vi "Vision Processing.vi"(4 "error in (no error)":errorcluster, 7 "Image Size":T1=enum."320x240") -> ()   [LabVIEW 2017]
doc: "This VI runs in parallel to other tasks. It gets images from the camera, processes them for color or shape and use that information to affect robot behavior."
uses:
  <vilib>/Rock Robotics/WPI/Camera/WPI_CameraImageSize.ctl
  <vilib>/Rock Robotics/WPI/Camera/WPI_CameraWhite Balance Values.ctl
  <vilib>/Rock Robotics/WPI/Camera/WPI_CameraExposure Values.ctl
  <vilib>/Rock Robotics/WPI/Camera/WPI_CameraFrameRate.ctl
  Robot Global Data.vi
  <vilib>/vision/NI_Vision_Development_Module.lvlib
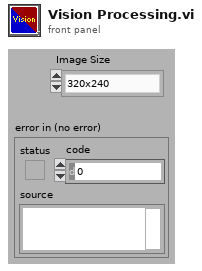
[diagram p1: front panel]
types:
  T1 = typedef "WPI_CameraImageSize.ctl" = enum16{"640x480", "320x240", "160x120", "Custom"}
  T2 = typedef "WPI_CameraFrameRate.ctl" = u32
  T3 = typedef "WPI_CameraExposure Values.ctl" = enum16{"Auto", "Flicker-free 50 Hz", "Flicker-free 60 Hz", "Hold current", "Custom"}
  T4 = typedef "WPI_CameraWhite Balance Values.ctl" = enum16{"Auto", "Fixed indoor", "Fixed outdoor 1", "Fixed outdoor 2", "Fixed fluorescent 1", "Fixed fluorescent 2", "Hold current", "Custom"}
  T5 = typedef "Image Type" = u32
  T6 = typedef "WPI_CameraDevRef.ctl" = cluster{"Camera Address":string, "CameraStatus":errorcluster}
  T7 = typedef "IMAQ Image.ctl" = refnum<image>
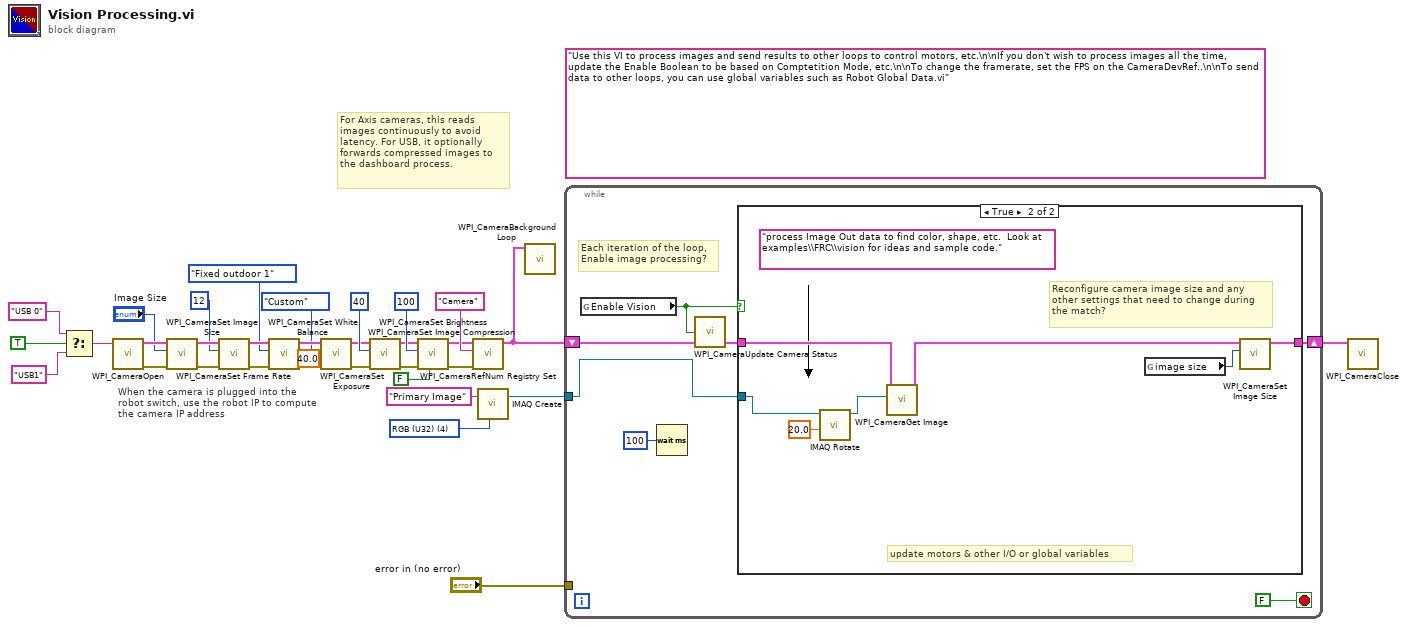
[diagram p0: block diagram]
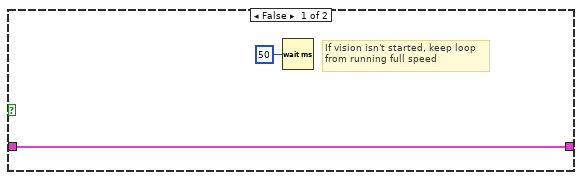
[diagram p2: hidden frame]
diagram:
  (unwired) "Use this VI to process images and send results to other loops to control motors, etc.\n\nIf you don't wish to process images all the time, update the Enable Boolean to be based on Comptetition Mode, etc.\n\nTo change the framerate, set the FPS on the CameraDevRef..\n\nTo send data to other loops, you can use global variables such as Robot Global Data.vi"
  w33 = T5 4 items=["Grayscale (U8)", "Grayscale (I16)", "Grayscale (SGL)", "Complex (CSG)", "RGB (U32)", "HSL (U32)", "RGB (U64)"] ("Image Type")
  # "When the camera is plugged into the\nrobot switch, use the robot IP to compute\nthe camera IP address"
  # "For Axis cameras, this reads\nimages continuously to avoid\nlatency. For USB, it optionally\nforwards compressed images to\nthe dashboard process."
  n1 = Select(t="USB 0" ("format string"), s=TRUE ("dot notation? (F)"), f="USB1" ("format string")) -> (s? t:f=w4:string)
  n2 = call <vilib>:"WPI_CameraOpen.vi"("Camera Address"=w4) -> ("error out"=w21:errorcluster, "CameraDevRef"=w22:T6)  [unwired: 1 in, 8 out]
  n3 = call <vilib>:"WPI_CameraSet Image Size.vi"("error in (no error)"=w21, "Image Size"="Image Size", "CameraDevRef"=w22) -> ("error out"=w20:errorcluster, "CameraDevRef Out"=w23:T6)  [unwired: 1 in, 6 out]
  n4 = call <vilib>:"WPI_CameraSet Frame Rate.vi"("error in (no error)"=w20, "Frame Rate (fps)"=T2 12, "CameraDevRef"=w23) -> ("error out"=w19:errorcluster, "CameraDevRef Out"=w25:T6)  [unwired: 7 out]
  n5 = call <vilib>:"WPI_CameraSet White Balance.vi"("error in (no error)"=w19, "White Balance"=WPI_CameraWhite_Balance_Values."Fixed outdoor 1", "CameraDevRef"=w25) -> ("error out"=w18:errorcluster, "CameraDevRef Out"=w24:T6)  [unwired: 1 in, 6 out]
  n6 = call <vilib>:"WPI_CameraSet Exposure.vi"("error in (no error)"=w18, "Exposure (%)"=40.0, "Exposure"=WPI_CameraExposure_Values."Custom", "CameraDevRef"=w24) -> ("error out"=w17:errorcluster, "CameraDevRef Out"=w27:T6)  [unwired: 6 out]
  n7 = call <vilib>:"WPI_CameraSet Image Compression.vi"("error in (no error)"=w17, "Compression"=40, "CameraDevRef"=w27) -> ("error out"=w16:errorcluster, "CameraDevRef Out"=w26:T6)  [unwired: 7 out]
  n8 = call <vilib>:"WPI_CameraSet Brightness.vi"("Force"=FALSE, "error in (no error)"=w16, "Brightness"=100, "CameraDevRef"=w26) -> ("error out"=w14:errorcluster, "CameraDevRef Out"=w15:T6)  [unwired: 6 out]
  n9 = call <vilib>:"WPI_CameraRefNum Registry Set.vi"("error in (no error)"=w14, "refnum name"="Camera", "CameraDevRef"=w15) -> ("CameraDevRef"=w10:T6)  [unwired: 1 in, 7 out]
  n10 = call "IMAQ Create"("Image Name"="Primary Image", "Image Type"=w33) -> ("New Image"=w31:T7)  [unwired: 2 in, 2 out]
  n11 = call <vilib>:"WPI_CameraBackground Loop.vi"("CameraDevRef"=w10) -> ()  [unwired: 11 in]
  n12 = while {
    shift-right: [w39] -> w8
    shift-left: w10 -> [w38]
    tunnel: w31 -> [w35]
    tunnel: "error in (no error)" -> [_]
    stop <- FALSE stop-if-true
    # "Each iteration of the loop,\nEnable image processing?"
    n13 = global read "Robot Global Data.vi" "Enable Vision"() -> (w36:bool)
    n14 = Wait (ms)(milliseconds to wait=u32 100) -> ()  [unwired: 1 out]
    n15 = call <vilib>:"WPI_CameraUpdate Camera Status.vi"("CameraDevRef In"=w38, "Enable Vision"=w36) -> ("CameraDevRef Out"=w37:T6)  [unwired: 3 in]
    n16 = case shown="True" w36 {
      tunnel: w35 -> [_ w45]
      tunnel: [w42 w49] -> w39
      tunnel: w37 -> [w42 w47]
      frame False {
        # "If vision isn't started, keep loop\nfrom running full speed"
        n17 = Wait (ms)(milliseconds to wait=u32 50) -> ()  [unwired: 1 out]
      }
      frame True {
        (unwired) "process Image Out data to find color, shape, etc.  Look at examples\\FRC\\vision for ideas and sample code."
        # "update motors & other I/O or global variables"
        # "Reconfigure camera image size and any\nother settings that need to change during\nthe match?"
        n18 = call "IMAQ Rotate"("Angle (degrees)"=sgl 20.0, "Image Src"=w45) -> ("Image Dst Out"=w44:T7)  [unwired: 8 in, 1 out]
        n19 = call <vilib>:"WPI_CameraGet Image.vi"("Image"=w44, "CameraDevRef"=w47) -> ("CameraDevRef Out"=w46:T6)  [unwired: 1 in, 8 out]
        n20 = global read "Robot Global Data.vi" "image size"() -> (w48:T1)
        n21 = call <vilib>:"WPI_CameraSet Image Size.vi"("Image Size"=w48, "CameraDevRef"=w46) -> ("CameraDevRef Out"=w49:T6)  [unwired: 2 in, 7 out]
      }
    }
  }
  n22 = call <vilib>:"WPI_CameraClose.vi"("CameraDevRef"=w8) -> ()  [unwired: 1 in, 10 out]
